vi "Get ControlRef from ctrlVI.vi"(8 "error in (no error)":errorcluster, 11 "VI ref in":refnum<vi>) -> (0 "error out":errorcluster, 2 "Control ref out":refnum<vi>, 3 "VI ref out":refnum<vi>)   [LabVIEW 2019, in "gRPC Scripting Tools.lvlib"]
uses:
  gRPC Scripting Tools.lvlib
  <vilib>/Utility/traverseref.llb/TRef TravTarget.ctl
  <vilib>/Utility/traverseref.llb/VI Scripting - Traverse.lvlib
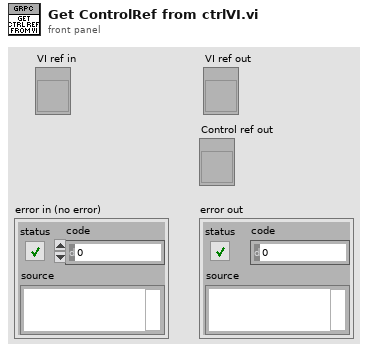
[diagram p1: front panel]
types:
  T1 = typedef "TRef TravTarget.ctl" = enum16{"FP", "BD", "Other"}
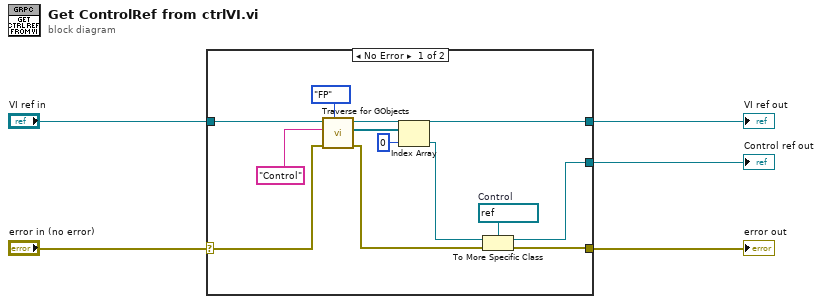
[diagram p0: block diagram]
diagram:
  n1 = case shown="No Error" "error in (no error)" {
    selector: "error in (no error)" -> [w10 w18]
    tunnel: "VI ref in" -> [w16 w19]
    tunnel: [w7 w18] -> w4
    tunnel: [w15 w19] -> w3
    tunnel: [w6 _] -> w1
    frame No Error {
      w9 = refnum<vi> refnum  # Control
      n2 = call <vilib>:"Traverse for GObjects.vi"("Traverse Target"=TRef_TravTarget."FP", "error in (no error)"=w10, "Class Name"="Control", "VI Refnum"=w16) -> ("error out"=w8:errorcluster, "References"=w14:refnum<vi>[], "dup VI Refnum"=w15:refnum<vi>)  [unwired: 4 in, 1 out]
      n3 = Index Array(array=w14, index=0) -> (element=w12:refnum<vi>)
      n4 = To More Specific Class(target class=w9, reference=w12, error in=w8) -> (specific class reference=w6:refnum<vi>, error out=w7:errorcluster)
    }
    frame Error {
    }
  }
  "error out" <- w4
  "Control ref out" <- w1
  "VI ref out" <- w3
